vi "Read Limited Functional.vi"(8 "error in (no error)":errorcluster, 11 "Test Selector in":refnum<class "Test Selector.lvclass">) -> (0 "error out":errorcluster, 2 "Limited Functional":bool[](array[boolean]), 3 "Test Selector out":refnum<class "Test Selector.lvclass">)   [LabVIEW 2019, in "Test Selector.lvlib" / "Test Selector.lvclass"]
uses:
  Test Selector.lvclass
  Test Selector.lvclass/Test Selector.ctl
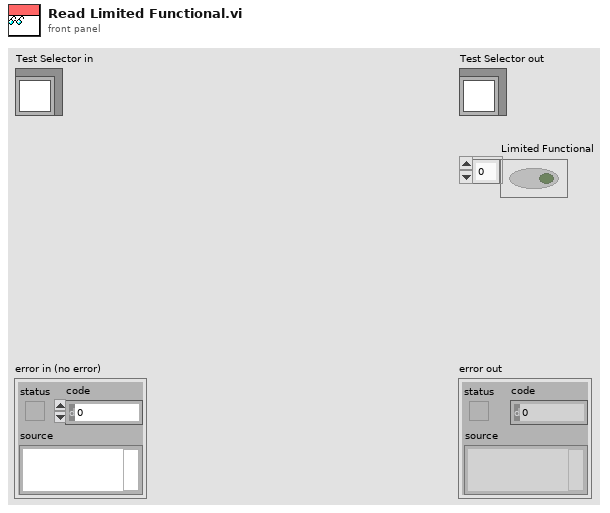
[diagram p1: front panel]
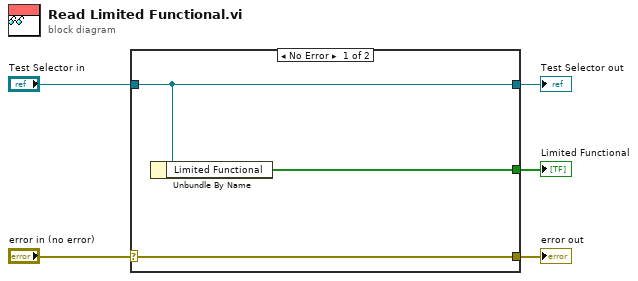
[diagram p0: block diagram]
diagram:
  n1 = case shown="No Error" "error in (no error)" {
    selector: "error in (no error)" -> [w8 w9]
    tunnel: [w8 w9] -> w4
    tunnel: [w7 w10] -> w2
    tunnel: "Test Selector in" -> [w7 w10]
    tunnel: [w6 _] -> w1
    frame No Error {
      n2 = Unbundle By Name(w7) -> ("Limited Functional"=w6:bool[])
    }
    frame Error {
    }
  }
  "error out" <- w4
  "Test Selector out" <- w2
  "Limited Functional" <- w1
